vi "Teleop.vi"(10 "Match Info":T1={"Autonomous Elapsed Seconds"=0.0, "TeleOp Elapsed Seconds"=0.0, "Disabled Elapsed Seconds"=0.0, "Visited Autonomous"=FALSE, "Visited TeleOp"=FALSE, "Visited Disabled"=FALSE, "Autonomous Settings"={"Autonomous Style"=enum."Independent", "VI Refnum"=refnum}}, 11 "Call Context":T2) -> ()   [LabVIEW 2013]
doc: "This VI is called for each TeleOp packet received from the DS where the robot is not disabled. It is often used to read from the joysticks and update I/O or to update setpoints for timed control loops. It should complete and return within 20 milliseconds or it may miss DS packets."
uses:
  <vilib>/Rock Robotics/WPI/DriverStation/WPI_DriverStationDerivedRobotMode.ctl
  <vilib>/Rock Robotics/WPI/DriverStation/WPI_DriverStationMatch Info.ctl
  Robot Global Data.vi
  <vilib>/Rock Robotics/WPI/Joystick/WPI_JoystickGetSetRefNum.vi
panel:
  in  "HarvSpeed":dbl=0.5
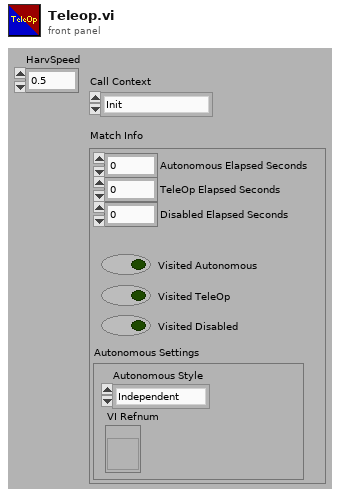
[diagram p1: front panel]
types:
  T1 = typedef "WPI_DriverStationMatch Info.ctl" = cluster{"Autonomous Elapsed Seconds":dbl, "TeleOp Elapsed Seconds":dbl, "Disabled Elapsed Seconds":dbl, "Visited Autonomous":bool, "Visited TeleOp":bool, "Visited Disabled":bool, "Autonomous Settings":cluster{"Autonomous Style":enum16{"Iterative", "Independent"}, "VI Refnum":refnum<vi>}}
  T2 = typedef "WPI_DriverStationDerivedRobotMode.ctl" = enum16{"Init", "Execute", "Stop"}
  T3 = typedef "WPI_JoystickDevRef.ctl" = cluster{"Device":T4}
  T4 = typedef "WPI_JoystickDeviceEnum.ctl" = enum16{"USB 1", "USB 2", "USB 3", "USB 4", "Kinect 1", "Kinect 2"}
  T5 = cluster{"axis 1 (x)":dbl, "axis 2 (y)":dbl, "axis 3 (throttle)":dbl, "axis 4":dbl, "axis 5":dbl, "axis 6":dbl}
  T6 = typedef "WPI_MotorControlDeviceRef.ctl" = cluster{"DeviceStatus":errorcluster, "Type":enum16{"PWM", "CAN"}, "PWM":cluster{"Digital Module":T7, "PWM Channel":T8, "DeadBand":T9}, "CAN":cluster{"Device Number":u8, "Control Mode":T10, "Semaphore":T11, "Max Vout":dbl}, "Invert":bool, "TransformRef":T12, "InvTransformRef":T12}
  T7 = typedef "FPGA_TypedefDigitalModule.ctl" = enum16{"Digital Module 1", "Digital Module 2"}
  T8 = typedef "FPGA_DIOPWMChannel.ctl" = enum8{"PWM 1", "PWM 2", "PWM 3", "PWM 4", "PWM 5", "PWM 6", "PWM 7", "PWM 8", "PWM 9", "PWM 10", "Invalid"}
  T9 = typedef "WPI_PWMDeadband.ctl" = cluster{"Name":string, "maxPositivePwm":i32, "minPositivePwm":i32, "centerPwm":i32, "maxNegativePwm":i32, "minNegativePwm":i32, "angularRange":u16}
  T10 = typedef "WPI_CANJaguar_ControlMode.ctl" = enum8{"Percent VBus", "Current", "Speed", "Position", "Voltage"}
  T11 = typedef "Semaphore RefNum" = refnum<k1>
  T12 = typedef "WPI_PWMTransform_ConPane.ctl" = refnum<vi>
  T13 = cluster{"Driver Station Digital Input (1-8)[0]":bool, "Driver Station Digital Input (1-8)[1]":bool, "Driver Station Digital Input (1-8)[2]":bool, "Driver Station Digital Input (1-8)[3]":bool, "Driver Station Digital Input (1-8)[4]":bool, "Driver Station Digital Input (1-8)[5]":bool, "Driver Station Digital Input (1-8)[6]":bool, "Driver Station Digital Input (1-8)[7]":bool, "Driver Station Digital Input (1-8)[8]":bool}
  T14 = typedef "WPI_JoystickButtonState.ctl" = cluster{"Button 1":bool, "Button 2":bool, "Button 3":bool, "Button 4":bool, "Button 5":bool, "Button 6":bool, "Button 7":bool, "Button 8":bool, "Button 9":bool, "Button 10":bool, "Button 11":bool, "Button 12":bool}
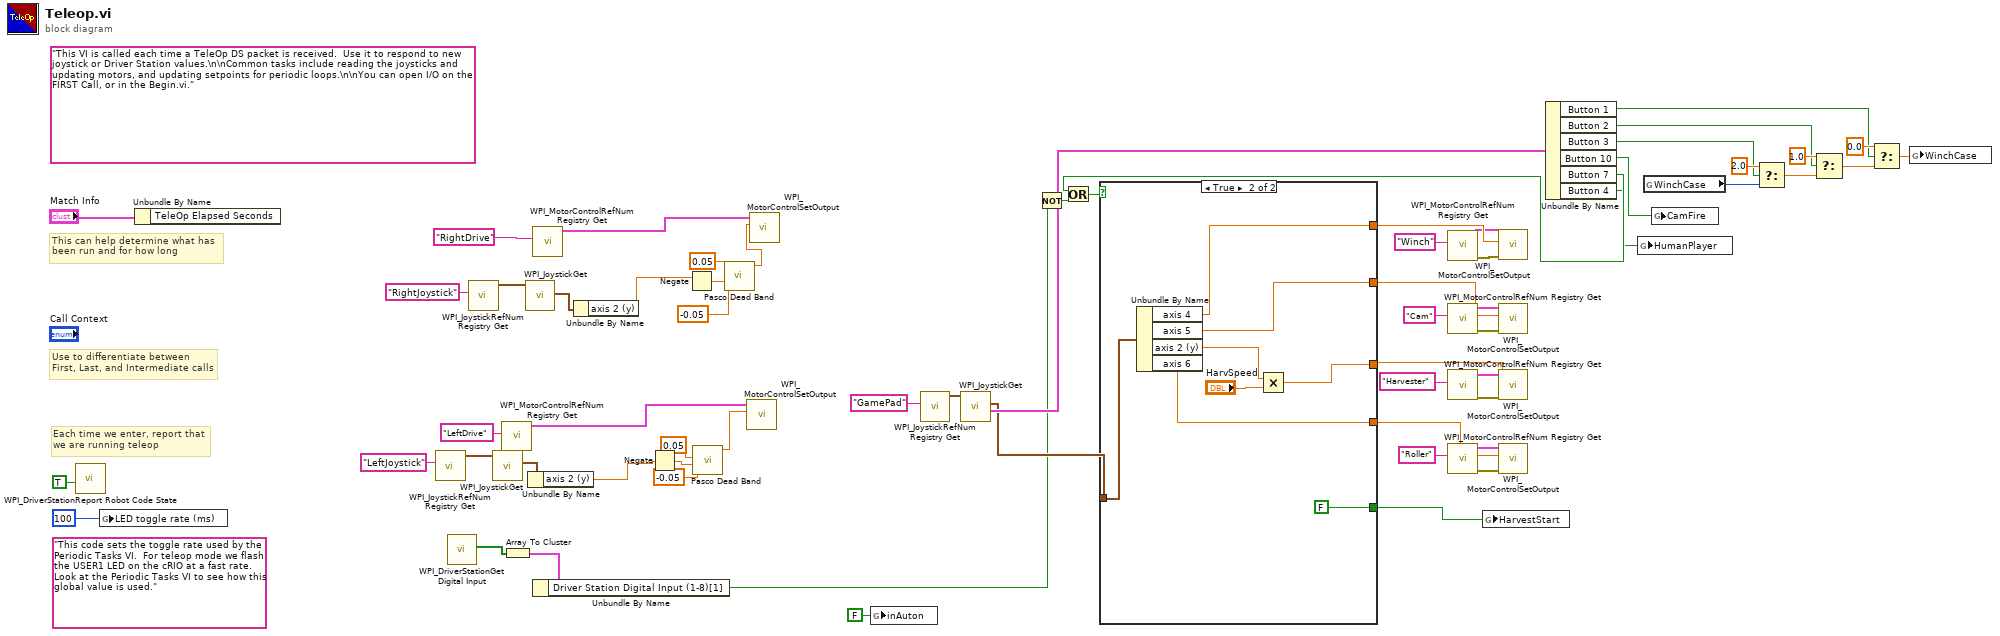
[diagram p0: block diagram]
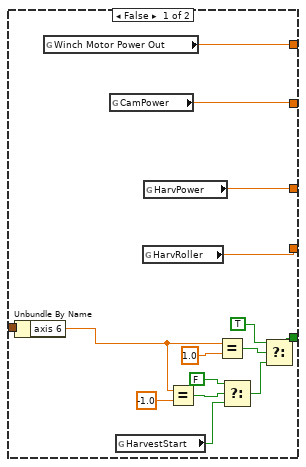
[diagram p2: hidden frame]
diagram:
  (unwired) "This code sets the toggle rate used by the Periodic Tasks VI.  For teleop mode we flash the USER1 LED on the cRIO at a fast rate.  Look at the Periodic Tasks VI to see how this global value is used."
  (unwired) "This VI is called each time a TeleOp DS packet is received.  Use it to respond to new joystick or Driver Station values.\n\nCommon tasks include reading the joysticks and updating motors, and updating setpoints for periodic loops.\n\nYou can open I/O on the FIRST Call, or in the Begin.vi."
  # "Each time we enter, report that\nwe are running teleop"
  # "Use to differentiate between\nFirst, Last, and Intermediate calls"
  # "This can help determine what has\nbeen run and for how long"
  n1 = call <vilib>:"WPI_DriverStationReport Robot Code State.vi"("TeleOp"=TRUE ("Autonomous")) -> ()  [unwired: 10 in, 1 out]
  n2 = global write "Robot Global Data.vi" "LED toggle rate (ms)"(u32 100 ("LED ms toggle rate")) -> ()
  n3 = Unbundle By Name("Match Info") -> ()  [unwired: 1 out]
  n4 = call <vilib>:"WPI_JoystickRefNum Registry Get.vi"("refnum name"="LeftJoystick") -> ("JoystickDevRef"=w52:T3)  [unwired: 9 in, 1 out]
  n5 = call <vilib>:"WPI_DriverStationGet Digital Input.vi"() -> ("Driver Station Digital Input (1-8)"=w6:bool[])  [unwired: 11 in]
  n6 = call <vilib>:"WPI_JoystickRefNum Registry Get.vi"("refnum name"="RightJoystick") -> ("JoystickDevRef"=w57:T3)  [unwired: 9 in, 1 out]
  n7 = call <vilib>:"WPI_JoystickGet.vi"("JoystickDevRef"=w52) -> ("Axes"=w51:T5)  [unwired: 4 in, 2 out]
  n8 = call <vilib>:"WPI_MotorControlRefNum Registry Get.vi"("refnum name"="LeftDrive") -> ("MotorControlDevRef"=w55:T6)  [unwired: 9 in, 1 out]
  n9 = Array To Cluster(array=w6) -> (cluster=w5:T13)
  n10 = call <vilib>:"WPI_JoystickGet.vi"("JoystickDevRef"=w57) -> ("Axes"=w56:T5)  [unwired: 4 in, 2 out]
  n11 = Unbundle By Name(w51) -> ("axis 2 (y)"=w50:dbl)
  n12 = call <vilib>:"WPI_MotorControlRefNum Registry Get.vi"("refnum name"="RightDrive") -> ("MotorControlDevRef"=w60:T6)  [unwired: 9 in, 1 out]
  n13 = Unbundle By Name(w5) -> ("Driver Station Digital Input (1-8)[1]"=w4:bool)
  n14 = Unbundle By Name(w56) -> ("axis 2 (y)"=w49:dbl)
  n15 = Negate(x=w50) -> (-x=w44:dbl)
  n16 = Negate(x=w49) -> (-x=w48:dbl)
  n17 = call "Pasco Dead Band.vi"("lower limit"=-0.05, "PWM Power"=w44, "upper limit"=0.05) -> ("PWM Power"=w41:dbl)  [unwired: 7 in, 1 out]
  n18 = call "Pasco Dead Band.vi"("lower limit"=-0.05, "PWM Power"=w48, "upper limit"=0.05) -> ("PWM Power"=w47:dbl)  [unwired: 7 in, 1 out]
  n19 = call <vilib>:"WPI_MotorControlSetOutput.vi"("Output"=w41, "MotorControlDevRef"=w55) -> ()  [unwired: 7 in, 3 out]
  n20 = call <vilib>:"WPI_MotorControlSetOutput.vi"("Output"=w47, "MotorControlDevRef"=w60) -> ()  [unwired: 7 in, 3 out]
  n21 = global write "Robot Global Data.vi" "inAuton"(FALSE ("inAuton")) -> ()
  n22 = call <vilib>:"WPI_JoystickRefNum Registry Get.vi"("refnum name"="GamePad") -> ("JoystickDevRef"=w39:T3)  [unwired: 9 in, 1 out]
  n23 = call <vilib>:"WPI_JoystickGet.vi"("JoystickDevRef"=w39) -> ("Buttons"=w12:T14, "Axes"=w10:T5)  [unwired: 4 in, 1 out]
  n24 = Not(x=w4) -> (.not. x?=w3:bool)
  n25 = call <vilib>:"WPI_MotorControlRefNum Registry Get.vi"("refnum name"="Winch") -> ("error out"=w30:errorcluster, "MotorControlDevRef"=w24:T6)  [unwired: 9 in]
  n26 = call <vilib>:"WPI_MotorControlRefNum Registry Get.vi"("refnum name"="Cam") -> ("error out"=w29:errorcluster, "MotorControlDevRef"=w28:T6)  [unwired: 9 in]
  n27 = call <vilib>:"WPI_MotorControlRefNum Registry Get.vi"("refnum name"="Harvester") -> ("error out"=w34:errorcluster, "MotorControlDevRef"=w33:T6)  [unwired: 9 in]
  n28 = call <vilib>:"WPI_MotorControlRefNum Registry Get.vi"("refnum name"="Roller") -> ("error out"=w36:errorcluster, "MotorControlDevRef"=w37:T6)  [unwired: 9 in]
  n29 = Unbundle By Name(w12) -> ("Button 1"=w15:bool, "Button 2"=w16:bool, "Button 3"=w17:bool, "Button 10"=w11:bool, "Button 7"=w7:bool, "Button 4"=w1:bool)
  n30 = Or(x=w7, y=w3) -> (x .or. y?=w8:bool)
  n31 = case shown="True" w8 {
    tunnel: [w78 w79] -> w35
    tunnel: [w77 w81] -> w31
    tunnel: w10 -> [w65 w86]
    tunnel: [w75 w85] -> w25
    tunnel: [w76 w84] -> w23
    tunnel: [w64 FALSE ("HarvestStart")] -> w9
    frame False {
      n32 = Unbundle By Name(w65) -> ("axis 6"=w73:dbl)
      n33 = global read "Robot Global Data.vi" "Winch Motor Power Out"() -> (w75:dbl)
      n34 = global read "Robot Global Data.vi" "CamPower"() -> (w76:dbl)
      n35 = global read "Robot Global Data.vi" "HarvestStart"() -> (w74:bool)
      n36 = global read "Robot Global Data.vi" "HarvRoller"() -> (w78:dbl)
      n37 = global read "Robot Global Data.vi" "HarvPower"() -> (w77:dbl)
      n38 = Equal?(x=w73, y=-1.0) -> (x = y?=w72:bool)
      n39 = Equal?(x=w73, y=1.0) -> (x = y?=w67:bool)
      n40 = Select(t=FALSE, s=w72, f=w74) -> (s? t:f=w70:bool)
      n41 = Select(t=TRUE, s=w67, f=w70) -> (s? t:f=w64:bool)
    }
    frame True {
      n42 = Unbundle By Name(w86) -> ("axis 4"=w85:dbl, "axis 5"=w84:dbl, "axis 2 (y)"=w82:dbl, "axis 6"=w79:dbl)
      n43 = Multiply(x=w82, y="HarvSpeed") -> (x*y=w81:dbl)
    }
  }
  n44 = global write "Robot Global Data.vi" "HarvestStart"(w9) -> ()
  n45 = call <vilib>:"WPI_MotorControlSetOutput.vi"("error in (no error)"=w30, "Output"=w25, "MotorControlDevRef"=w24) -> ()  [unwired: 6 in, 3 out]
  n46 = call <vilib>:"WPI_MotorControlSetOutput.vi"("error in (no error)"=w29, "Output"=w23, "MotorControlDevRef"=w28) -> ()  [unwired: 6 in, 3 out]
  n47 = call <vilib>:"WPI_MotorControlSetOutput.vi"("error in (no error)"=w34, "Output"=w31, "MotorControlDevRef"=w33) -> ()  [unwired: 6 in, 3 out]
  n48 = call <vilib>:"WPI_MotorControlSetOutput.vi"("error in (no error)"=w36, "Output"=w35, "MotorControlDevRef"=w37) -> ()  [unwired: 6 in, 3 out]
  n49 = global write "Robot Global Data.vi" "HumanPlayer"(w1) -> ()
  n50 = global read "Robot Global Data.vi" "WinchCase"() -> (w13:i32)
  n51 = global write "Robot Global Data.vi" "CamFire"(w11) -> ()
  n52 = Select(t=2.0, s=w17, f=w13) -> (s? t:f=w22:dbl)
  n53 = Select(t=1.0, s=w16, f=w22) -> (s? t:f=w21:dbl)
  n54 = Select(t=0.0, s=w15, f=w21) -> (s? t:f=w14:dbl)
  n55 = global write "Robot Global Data.vi" "WinchCase"(w14) -> ()
